vi "Insert placeholder data to publish .vi"(8 "error in (no error)":errorcluster, 10 "Measured_Data":dbl[](array[numeric]), 11 "Publishable IDs":string[](array[string])) -> (0 "error out":errorcluster, 3 "Array":dbl[](array[numeric]))   [LabVIEW 2013]
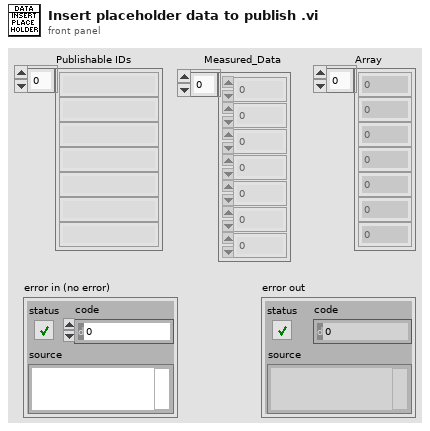
[diagram p1: front panel]
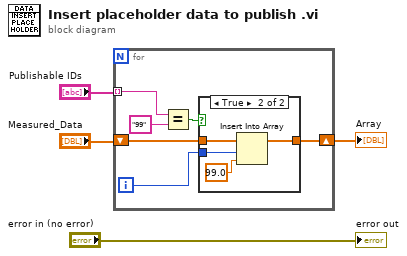
[diagram p0: block diagram]
diagram:
  n1 = for {
    tunnel: "Publishable IDs" -> [w10] mode=indexing
    shift-right: [w7] -> w4
    shift-left: "Measured_Data" -> [w8]
    i -> [w6]
    n2 = Equal?(x=w10, y="99") -> (x = y?=w5:bool)
    n3 = case shown="True" w5 {
      tunnel: w8 -> [w11 w15]
      tunnel: [w11 w14] -> w7
      tunnel: w6 -> [_ w13]
      frame False {
      }
      frame True {
        n4 = Insert Into Array(array=w15, index=w13, new element=99.0 ("new element/subarray")) -> (w14:dbl[])
      }
    }
  }
  "Array" <- w4
  "error out" <- "error in (no error)"
